vi "Visa Read All.vi"(8 "error in (no error)":errorcluster, 11 "VISA resource name":refnum<visa-resource-name>) -> (0 "error out":errorcluster, 1 "Read Buffer":string, 3 "VISA resource name out":refnum<visa-resource-name>)   [LabVIEW 2014, in "Agilent U2000 Series.lvlib"]
doc: "Reads all data in the VISA buffer."
uses:
  Agilent U2000 Series.lvlib
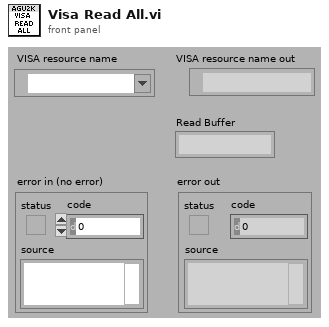
[diagram p1: front panel]
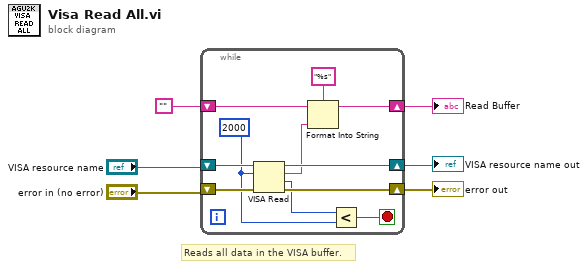
[diagram p0: block diagram]
diagram:
  # "Reads all data in the VISA buffer."
  n1 = while {
    shift-right: [w14] -> w2
    shift-left: "error in (no error)" -> [w16]
    shift-right: [w15] -> w3
    shift-left: "VISA resource name" -> [w17]
    shift-right: [w7] -> w1
    shift-left: "" -> [w9]
    stop <- w11 stop-if-true
    w12 = u32 2000 ("byte count")
    n2 = VISA Read(VISA resource name=w17, byte count=w12, error in (no error)=w16) -> (VISA resource name out=w15:refnum<visa-resource-name>, read buffer=w8:string, return count=w13:u32, error out=w14:errorcluster)
    n3 = Format Into String(format string="%s", initial string=w9, w8) -> (resulting string=w7:string)  [unwired: 1 in, 1 out]
    n4 = Less?(x=w13, y=w12) -> (x < y?=w11:bool)
  }
  "VISA resource name out" <- w3
  "error out" <- w2
  "Read Buffer" <- w1
